vi "CRYTest Changing State.vi"(6 "Save?":bool, 8 "Origine Calibration":T1 {"Calibration 2D"."Sens Curve"."Z data" items=["dB", "Lin"]; "Calibration 2D"."Sens Curve"."X data" items=["dB", "Lin"]; "Calibration 2D"."Sens Curve"."Y data" items=["dB", "Lin"]; "Calibration 2D"."Sens Curve"."Z dB ref" format="%.1f"; "Calibration 2D"."Sens Curve"."Z axis" items=["Log", "Lin"]; "Calibration 2D"."Sens Curve"."X dB ref" format="%.1f"; "Calibration 2D"."Sens Curve"."X axis" items=["Log", "Lin"]; "Calibration 2D"."Sens Curve"."Y axis" items=["Log", "Lin"]; "Calibration 2D"."Sens Curve"."Y dB ref" format="%.1f"; "Calibration 2D"."Sens Curve"."Curve"."z" format="%.2f"; "Calibration 2D"."Sens Curve"."Curve"."y" format="%.2p"; "Calibration 2D"."Sens Curve"."Curve"."x" format="%.2f"; "Calibration 2D"."EQ Curve"."Z data" items=["dB", "Lin"]; "Calibration 2D"."EQ Curve"."X data" items=["dB", "Lin"]; "Calibration 2D"."EQ Curve"."Y data" items=["dB", "Lin"]; "Calibration 2D"."EQ Curve"."Z dB ref" format="%.1f"; "Calibration 2D"."EQ Curve"."Z axis" items=["Log", "Lin"]; "Calibration 2D"."EQ Curve"."X dB ref" format="%.1f"; "Calibration 2D"."EQ Curve"."X axis" items=["Log", "Lin"]; "Calibration 2D"."EQ Curve"."Y axis" items=["Log", "Lin"]; "Calibration 2D"."EQ Curve"."Y dB ref" format="%.1f"; "Calibration 2D"."EQ Curve"."Curve"."z" format="%.2f"; "Calibration 2D"."EQ Curve"."Curve"."y" format="%.2f"; "Calibration 2D"."EQ Curve"."Curve"."x" format="%.2f"; "Calibration 2D"."Corr Curve"."Z data" items=["dB", "Lin"]; "Calibration 2D"."Corr Curve"."X data" items=["dB", "Lin"]; "Calibration 2D"."Corr Curve"."Y data" items=["dB", "Lin"]; "Calibration 2D"."Corr Curve"."Z dB ref" format="%.1f"; "Calibration 2D"."Corr Curve"."Z axis" items=["Log", "Lin"]; "Calibration 2D"."Corr Curve"."X dB ref" format="%.1f"; "Calibration 2D"."Corr Curve"."X axis" items=["Log", "Lin"]; "Calibration 2D"."Corr Curve"."Y axis" items=["Log", "Lin"]; "Calibration 2D"."Corr Curve"."Y dB ref" format="%.1f"; "Calibration 2D"."Corr Curve"."Curve"."z" format="%.2f"; "Calibration 2D"."Corr Curve"."Curve"."y" format="%.2f"; "Calibration 2D"."Corr Curve"."Curve"."x" format="%.2f"; "Calibration 2D"."Calibration"."EQ Step size" items=["R10", "R20", "R40", "R80", "User"]; "Calibration 2D"."Calibration"."Corr Step size" items=["R10", "R20", "R40", "R80", "User"]}, 9 "New Calibration":T1 {"Calibration 2D"."Sens Curve"."Z data" items=["dB", "Lin"]; "Calibration 2D"."Sens Curve"."X data" items=["dB", "Lin"]; "Calibration 2D"."Sens Curve"."Y data" items=["dB", "Lin"]; "Calibration 2D"."Sens Curve"."Z dB ref" format="%.1f"; "Calibration 2D"."Sens Curve"."Z axis" items=["Log", "Lin"]; "Calibration 2D"."Sens Curve"."X dB ref" format="%.1f"; "Calibration 2D"."Sens Curve"."X axis" items=["Log", "Lin"]; "Calibration 2D"."Sens Curve"."Y axis" items=["Log", "Lin"]; "Calibration 2D"."Sens Curve"."Y dB ref" format="%.1f"; "Calibration 2D"."Sens Curve"."Curve"."z" format="%.2f"; "Calibration 2D"."Sens Curve"."Curve"."y" format="%.2p"; "Calibration 2D"."Sens Curve"."Curve"."x" format="%.2f"; "Calibration 2D"."EQ Curve"."Z data" items=["dB", "Lin"]; "Calibration 2D"."EQ Curve"."X data" items=["dB", "Lin"]; "Calibration 2D"."EQ Curve"."Y data" items=["dB", "Lin"]; "Calibration 2D"."EQ Curve"."Z dB ref" format="%.1f"; "Calibration 2D"."EQ Curve"."Z axis" items=["Log", "Lin"]; "Calibration 2D"."EQ Curve"."X dB ref" format="%.1f"; "Calibration 2D"."EQ Curve"."X axis" items=["Log", "Lin"]; "Calibration 2D"."EQ Curve"."Y axis" items=["Log", "Lin"]; "Calibration 2D"."EQ Curve"."Y dB ref" format="%.1f"; "Calibration 2D"."EQ Curve"."Curve"."z" format="%.2f"; "Calibration 2D"."EQ Curve"."Curve"."y" format="%.2f"; "Calibration 2D"."EQ Curve"."Curve"."x" format="%.2f"; "Calibration 2D"."Corr Curve"."Z data" items=["dB", "Lin"]; "Calibration 2D"."Corr Curve"."X data" items=["dB", "Lin"]; "Calibration 2D"."Corr Curve"."Y data" items=["dB", "Lin"]; "Calibration 2D"."Corr Curve"."Z dB ref" format="%.1f"; "Calibration 2D"."Corr Curve"."Z axis" items=["Log", "Lin"]; "Calibration 2D"."Corr Curve"."X dB ref" format="%.1f"; "Calibration 2D"."Corr Curve"."X axis" items=["Log", "Lin"]; "Calibration 2D"."Corr Curve"."Y axis" items=["Log", "Lin"]; "Calibration 2D"."Corr Curve"."Y dB ref" format="%.1f"; "Calibration 2D"."Corr Curve"."Curve"."z" format="%.2f"; "Calibration 2D"."Corr Curve"."Curve"."y" format="%.2f"; "Calibration 2D"."Corr Curve"."Curve"."x" format="%.2f"; "Calibration 2D"."Calibration"."EQ Step size" items=["R10", "R20", "R40", "R80", "User"]; "Calibration 2D"."Calibration"."Corr Step size" items=["R10", "R20", "R40", "R80", "User"]}, 10 "Signal Type":string, 11 "In/Out?":bool) -> (1 "Calibration 2D Cluster":T2={"Calibration"={"Calibration Step Name"="", "Device"="", "Correction Curve Name"="", "Equalization Curve Name"="", "Sensitivity Curve Name"="", "Corr Folder and File"="", "EQ Folder and File"="", "Sens Folder and File"="", "Corr Step size"=0, "EQ Step size"=0, "Input"=FALSE, "Last Cal Date (sec)"=timestamp(0 s since 1904-01-01), "Cha Name"="", "Corr Curve Found"=FALSE, "EQ Curve Found"=FALSE, "Sens Curve Found"=FALSE, "Signal Type"="", "Calibrated Device"="", "Hz"=0}, "Corr Curve"={"Name"="", "Curve"=[], "X data"=1, "Y data"=1, "Z data"=1, "X axis"=0, "Y axis"=1, "Z axis"=1, "X unit"="Hz", "Y unit"="", "Z unit"="deg.", "X dB ref"=1.0, "Y dB ref"=1.0, "Z dB ref"=1.0, "single val"=FALSE, "protected"=FALSE, "display X"=TRUE, "display Y"=TRUE, "display Z"=TRUE, "Test Info"="", "Step No."=0, "Plot Settings"={"Color"=0, "Interpolation"=0, "Point Style"=0, "Line Style"=0, "Point Color"=0, "Line Width"=0, "Bar Plot Style"=0, "Fill To"=0}, "AutoProtect"=FALSE}, "EQ Curve"={"Name"="", "Curve"=[], "X data"=1, "Y data"=1, "Z data"=1, "X axis"=0, "Y axis"=1, "Z axis"=1, "X unit"="Hz", "Y unit"="", "Z unit"="deg.", "X dB ref"=1.0, "Y dB ref"=1.0, "Z dB ref"=1.0, "single val"=FALSE, "protected"=FALSE, "display X"=TRUE, "display Y"=TRUE, "display Z"=TRUE, "Test Info"="", "Step No."=0, "Plot Settings"={"Color"=0, "Interpolation"=0, "Point Style"=0, "Line Style"=0, "Point Color"=0, "Line Width"=0, "Bar Plot Style"=0, "Fill To"=0}, "AutoProtect"=FALSE}, "Sens Curve"={"Name"="", "Curve"=[], "X data"=1, "Y data"=1, "Z data"=1, "X axis"=0, "Y axis"=1, "Z axis"=1, "X unit"="Hz", "Y unit"="", "Z unit"="deg.", "X dB ref"=1.0, "Y dB ref"=1.0, "Z dB ref"=1.0, "single val"=FALSE, "protected"=FALSE, "display X"=TRUE, "display Y"=TRUE, "display Z"=TRUE, "Test Info"="", "Step No."=0, "Plot Settings"={"Color"=0, "Interpolation"=0, "Point Style"=0, "Line Style"=0, "Point Color"=0, "Line Width"=0, "Bar Plot Style"=0, "Fill To"=0}, "AutoProtect"=FALSE}} {"Sens Curve"."Z data" items=["dB", "Lin"]; "Sens Curve"."X data" items=["dB", "Lin"]; "Sens Curve"."Y data" items=["dB", "Lin"]; "Sens Curve"."Z dB ref" format="%.1f"; "Sens Curve"."Z axis" items=["Log", "Lin"]; "Sens Curve"."X dB ref" format="%.1f"; "Sens Curve"."X axis" items=["Log", "Lin"]; "Sens Curve"."Y axis" items=["Log", "Lin"]; "Sens Curve"."Y dB ref" format="%.1f"; "Sens Curve"."Curve"."z" format="%.2f"; "Sens Curve"."Curve"."y" format="%.2f"; "Sens Curve"."Curve"."x" format="%.2f"; "EQ Curve"."Z data" items=["dB", "Lin"]; "EQ Curve"."X data" items=["dB", "Lin"]; "EQ Curve"."Y data" items=["dB", "Lin"]; "EQ Curve"."Z dB ref" format="%.1f"; "EQ Curve"."Z axis" items=["Log", "Lin"]; "EQ Curve"."X dB ref" format="%.1f"; "EQ Curve"."X axis" items=["Log", "Lin"]; "EQ Curve"."Y axis" items=["Log", "Lin"]; "EQ Curve"."Y dB ref" format="%.1f"; "EQ Curve"."Curve"."z" format="%.2f"; "EQ Curve"."Curve"."y" format="%.2f"; "EQ Curve"."Curve"."x" format="%.2f"; "Corr Curve"."Z data" items=["dB", "Lin"]; "Corr Curve"."X data" items=["dB", "Lin"]; "Corr Curve"."Y data" items=["dB", "Lin"]; "Corr Curve"."Z dB ref" format="%.1f"; "Corr Curve"."Z axis" items=["Log", "Lin"]; "Corr Curve"."X dB ref" format="%.1f"; "Corr Curve"."X axis" items=["Log", "Lin"]; "Corr Curve"."Y axis" items=["Log", "Lin"]; "Corr Curve"."Y dB ref" format="%.1f"; "Corr Curve"."Curve"."z" format="%.2f"; "Corr Curve"."Curve"."y" format="%.2f"; "Corr Curve"."Curve"."x" format="%.2f"; "Calibration"."EQ Step size" items=["R10", "R20", "R40", "R80", "User"]; "Calibration"."Corr Step size" items=["R10", "R20", "R40", "R80", "User"]}, 2 "Changed/Added":bool, 3 "Index":i32)   [LabVIEW 2013]
uses:
  Typedef Control/CRYCalibration All Cluster.ctl
  Typedef Control/CRYCalibration 2DCluster.ctl
  Typedef Control/CRYCalibration Cluster.ctl
  Typedef Control/CRYData Cluster.ctl
  CRYProject/CRYProject Editor Global.vi
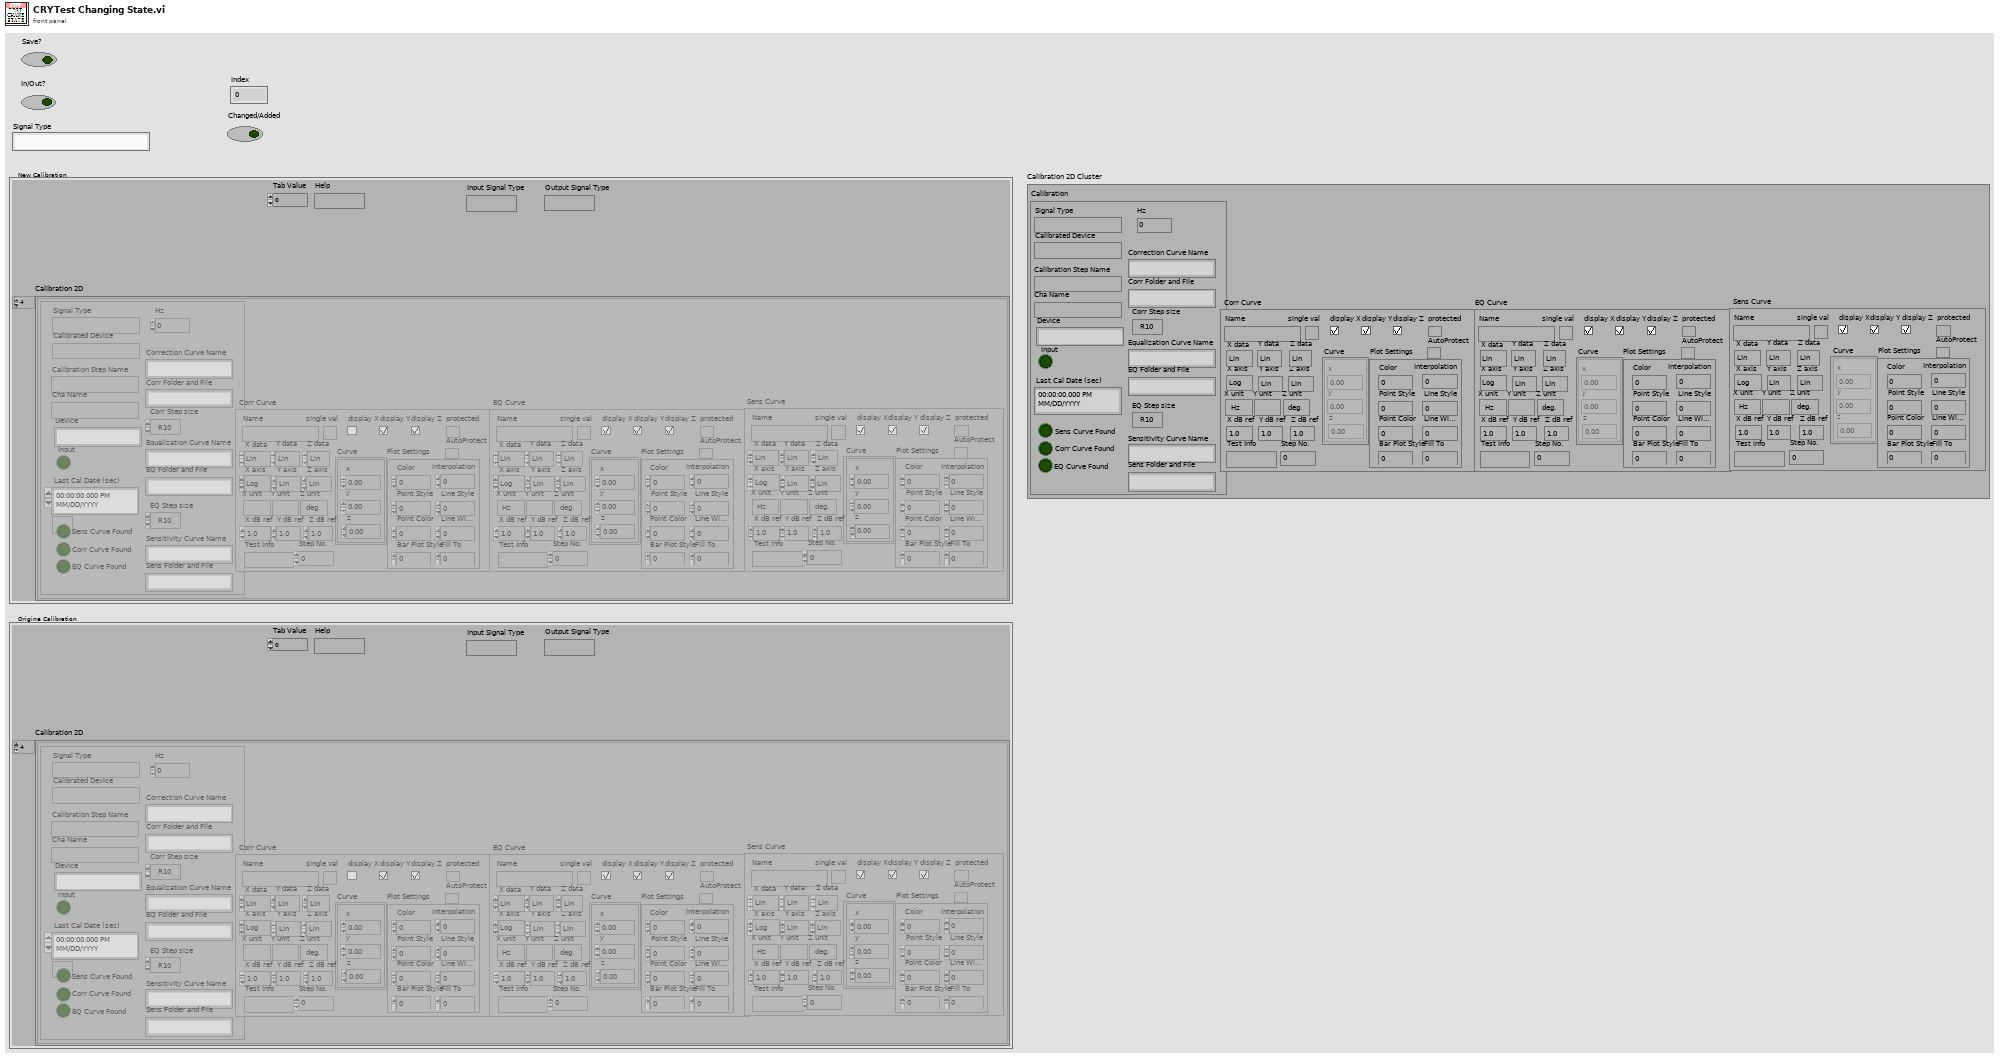
[diagram p1: front panel]
types:
  T1 = typedef "CRYCalibration All Cluster.ctl" = cluster{"Calibration 2D":T2[], "Help":string, "Tab Value":i32, "Input Signal Type":string, "Output Signal Type":string}
  T2 = typedef "CRYCalibration 2DCluster.ctl" = cluster{"Calibration":T3, "Corr Curve":T4, "EQ Curve":T4, "Sens Curve":T4}
  T3 = typedef "CRYCalibration Cluster.ctl" = cluster{"Calibration Step Name":string, "Device":string, "Correction Curve Name":string, "Equalization Curve Name":string, "Sensitivity Curve Name":string, "Corr Folder and File":string, "EQ Folder and File":string, "Sens Folder and File":string, "Corr Step size":u16, "EQ Step size":u16, "Input":bool, "Last Cal Date (sec)":timestamp, "Cha Name":string, "Corr Curve Found":bool, "EQ Curve Found":bool, "Sens Curve Found":bool, "Signal Type":string, "Calibrated Device":string, "Hz":u32}
  T4 = typedef "CRYData Cluster.ctl" = cluster{"Name":string, "Curve":cluster{"x":dbl, "y":dbl, "z":dbl}[], "X data":u16, "Y data":u16, "Z data":u16, "X axis":u16, "Y axis":u16, "Z axis":u16, "X unit":string, "Y unit":string, "Z unit":string, "X dB ref":dbl, "Y dB ref":dbl, "Z dB ref":dbl, "single val":bool, "protected":bool, "display X":bool, "display Y":bool, "display Z":bool, "Test Info":string, "Step No.":i32, "Plot Settings":cluster{"Color":u32, "Interpolation":u8, "Point Style":u8, "Line Style":u8, "Point Color":u32, "Line Width":u8, "Bar Plot Style":u8, "Fill To":i16}, "AutoProtect":bool}
  T5 = typedef "CRYStep.ctl" = cluster{"No.VI":i32, "Category":string, "StepName":string, "Seq setup flattened":string, "Comment":string, "Steps config.":bool[], "Jump config":i32[], "Start":dbl, "Increment":dbl, "Name":string, "Unit":string, "Y data":u16, "Y prefix":string, "Y dB ref":dbl, "Y unit":string, "Repeat State Array":cluster{"Start":dbl, "Increment":dbl, "Count":i32, "Num":i32}[]}
  T6 = cluster{"Calibration":cluster{"Calibration Step Name":bool, "Device":bool, "Correction Curve Name":bool, "Equalization Curve Name":bool, "Sensitivity Curve Name":bool, "Corr Folder and File":bool, "EQ Folder and File":bool, "Sens Folder and File":bool, "Corr Step size":bool, "EQ Step size":bool, "Input":bool, "Last Cal Date (sec)":bool, "Cha Name":bool, "Corr Curve Found":bool, "EQ Curve Found":bool, "Sens Curve Found":bool, "Signal Type":bool, "Calibrated Device":bool, "Hz":bool}, "Corr Curve":cluster{"Name":bool, "Curve":cluster{"x":bool, "y":bool, "z":bool}[], "X data":bool, "Y data":bool, "Z data":bool, "X axis":bool, "Y axis":bool, "Z axis":bool, "X unit":bool, "Y unit":bool, "Z unit":bool, "X dB ref":bool, "Y dB ref":bool, "Z dB ref":bool, "single val":bool, "protected":bool, "display X":bool, "display Y":bool, "display Z":bool, "Test Info":bool, "Step No.":bool, "Plot Settings":cluster{"Color":bool, "Interpolation":bool, "Point Style":bool, "Line Style":bool, "Point Color":bool, "Line Width":bool, "Bar Plot Style":bool, "Fill To":bool}, "AutoProtect":bool}, "EQ Curve":cluster{"Name":bool, "Curve":cluster{"x":bool, "y":bool, "z":bool}[], "X data":bool, "Y data":bool, "Z data":bool, "X axis":bool, "Y axis":bool, "Z axis":bool, "X unit":bool, "Y unit":bool, "Z unit":bool, "X dB ref":bool, "Y dB ref":bool, "Z dB ref":bool, "single val":bool, "protected":bool, "display X":bool, "display Y":bool, "display Z":bool, "Test Info":bool, "Step No.":bool, "Plot Settings":cluster{"Color":bool, "Interpolation":bool, "Point Style":bool, "Line Style":bool, "Point Color":bool, "Line Width":bool, "Bar Plot Style":bool, "Fill To":bool}, "AutoProtect":bool}, "Sens Curve":cluster{"Name":bool, "Curve":cluster{"x":bool, "y":bool, "z":bool}[], "X data":bool, "Y data":bool, "Z data":bool, "X axis":bool, "Y axis":bool, "Z axis":bool, "X unit":bool, "Y unit":bool, "Z unit":bool, "X dB ref":bool, "Y dB ref":bool, "Z dB ref":bool, "single val":bool, "protected":bool, "display X":bool, "display Y":bool, "display Z":bool, "Test Info":bool, "Step No.":bool, "Plot Settings":cluster{"Color":bool, "Interpolation":bool, "Point Style":bool, "Line Style":bool, "Point Color":bool, "Line Width":bool, "Bar Plot Style":bool, "Fill To":bool}, "AutoProtect":bool}}
  T7 = cluster{"Calibration Step Name":bool, "Device":bool, "Correction Curve Name":bool, "Equalization Curve Name":bool, "Sensitivity Curve Name":bool, "Corr Folder and File":bool, "EQ Folder and File":bool, "Sens Folder and File":bool, "Corr Step size":bool, "EQ Step size":bool, "Input":bool, "Last Cal Date (sec)":bool, "Cha Name":bool, "Corr Curve Found":bool, "EQ Curve Found":bool, "Sens Curve Found":bool, "Signal Type":bool, "Calibrated Device":bool, "Hz":bool}
  T8 = cluster{"Name":bool, "Curve":cluster{"x":bool, "y":bool, "z":bool}[], "X data":bool, "Y data":bool, "Z data":bool, "X axis":bool, "Y axis":bool, "Z axis":bool, "X unit":bool, "Y unit":bool, "Z unit":bool, "X dB ref":bool, "Y dB ref":bool, "Z dB ref":bool, "single val":bool, "protected":bool, "display X":bool, "display Y":bool, "display Z":bool, "Test Info":bool, "Step No.":bool, "Plot Settings":cluster{"Color":bool, "Interpolation":bool, "Point Style":bool, "Line Style":bool, "Point Color":bool, "Line Width":bool, "Bar Plot Style":bool, "Fill To":bool}, "AutoProtect":bool}
  T9 = cluster{"Name":bool, "Curve":cluster{"x":bool, "y":bool, "z":bool}[], "X data":bool, "Y data":bool, "Z data":bool, "X axis":bool, "Y axis":bool, "Z axis":bool, "X unit":bool, "Y unit":bool, "Z unit":bool, "X dB ref":bool, "Y dB ref":bool, "Z dB ref":bool, "single val":bool, "protected":bool, "display X":bool, "display Y":bool, "display Z":bool, "Test Info":bool, "Step No.":bool, "Plot Settings":cluster{"Color":bool, "Interpolation":bool, "Point Style":bool, "Line Style":bool, "Point Color":bool, "Line Width":bool, "Bar Plot Style":bool, "Fill To":bool}, "AutoProtect":bool}[]
  T10 = cluster{"Color":bool, "Interpolation":bool, "Point Style":bool, "Line Style":bool, "Point Color":bool, "Line Width":bool, "Bar Plot Style":bool, "Fill To":bool}
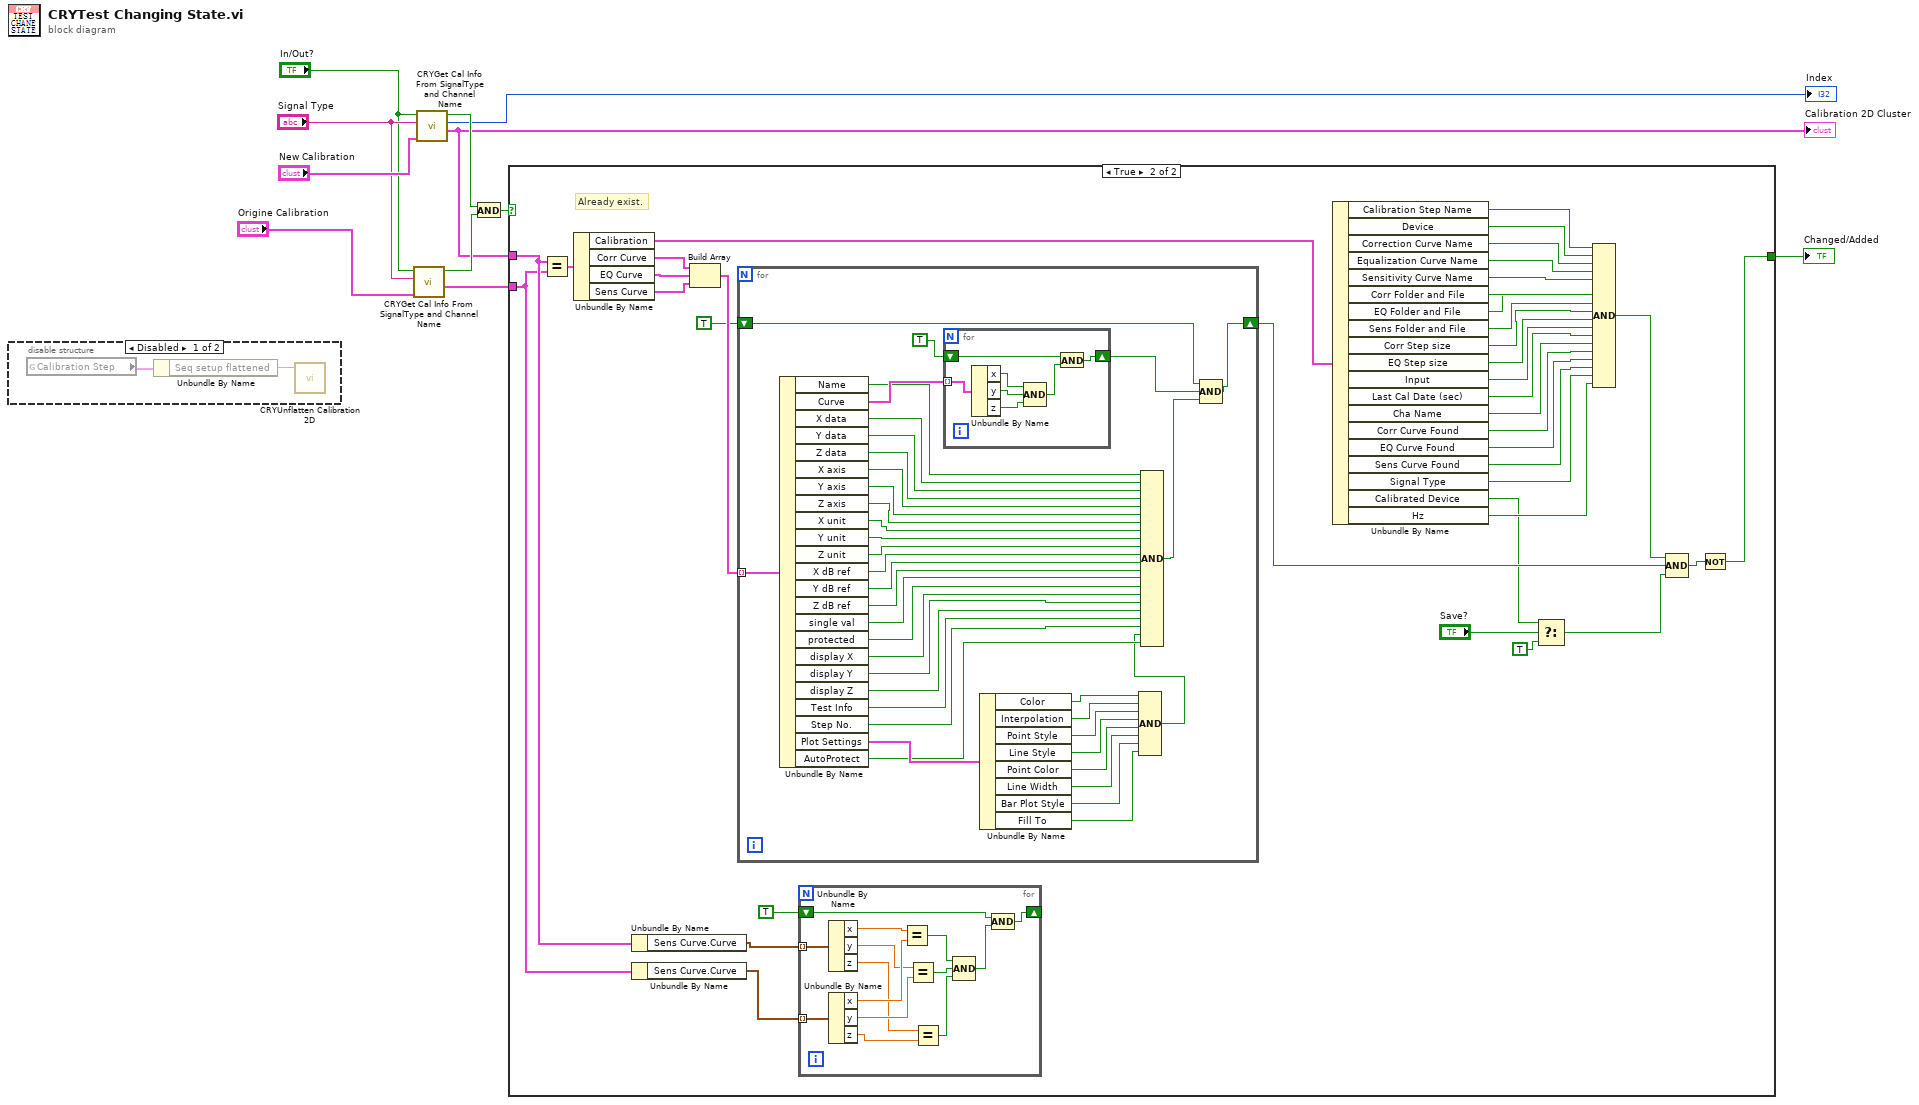
[diagram p0: block diagram]
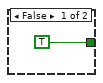
[diagram p3: hidden frame]
diagram:
  n1 = disable-structure shown="Disabled" {
    frame Disabled {
      n2 = global read "CRYProject Editor Global.vi" "Calibration Step"() -> (w13:T5)
      n3 = Unbundle By Name(w13) -> ("Seq setup flattened"=w12:string)
      n4 = call "CRYUnflatten Calibration 2D.vi"("Flattened Calibration"=w12) -> ()  [unwired: 8 in, 3 out]
    }
    frame Enabled {
    }
  }
  n5 = call "CRYGet Cal Info From SignalType and Channel Name.vi"("Calibration"="Origine Calibration", "Signal Type"="Signal Type", "In/Out?"="In/Out?") -> ("Calibration 2D Cluster"=w3:T2, "Exist"=w7:bool)  [unwired: 6 in, 1 out]
  n6 = call "CRYGet Cal Info From SignalType and Channel Name.vi"("Calibration"="New Calibration", "Signal Type"="Signal Type", "In/Out?"="In/Out?") -> ("Calibration 2D Cluster"=w2:T2, "Index"=→"Index":i32, "Exist"=w8:bool)  [unwired: 6 in]
  "Calibration 2D Cluster" <- w2
  n7 = And(x=w8, y=w7) -> (x .and. y?=w6:bool)
  n8 = case shown="True" w6 {
    tunnel: [TRUE ("Changed") w25] -> w5
    tunnel: w3 -> [_ w22]
    tunnel: w2 -> [_ w23]
    frame False {
    }
    frame True {
      # "Already exist."
      n9 = Equal?(x=w23, y=w22) -> (x = y?=w52:T6)
      n10 = Unbundle By Name(w52) -> ("Calibration"=w51:T7, "Corr Curve"=w50:T8, "EQ Curve"=w49:T8, "Sens Curve"=w24:T8)
      n11 = Unbundle By Name(w23) -> ("Sens Curve.Curve"=w21:cluster{"x":dbl, "y":dbl, "z":dbl}[])
      n12 = Unbundle By Name(w22) -> ("Sens Curve.Curve"=w20:cluster{"x":dbl, "y":dbl, "z":dbl}[])
      n13 = Build Array(w50, w49, w24) -> (w48:T9)
      n14 = for {
        tunnel: w48 -> [w104] mode=indexing
        shift-right: [w68] -> w27
        shift-left: TRUE ("Name") -> [w71]
        n15 = Unbundle By Name(w104) -> ("Name"=w100:bool, "Curve"=w103:cluster{"x":bool, "y":bool, "z":bool}[], "X data"=w99:bool, "Y data"=w98:bool, "Z data"=w97:bool, "X axis"=w96:bool, "Y axis"=w95:bool, "Z axis"=w94:bool, "X unit"=w93:bool, "Y unit"=w92:bool, "Z unit"=w91:bool, "X dB ref"=w90:bool, "Y dB ref"=w89:bool, "Z dB ref"=w88:bool, "single val"=w87:bool, "protected"=w86:bool, "display X"=w85:bool, "display Y"=w84:bool, "display Z"=w83:bool, "Test Info"=w82:bool, "Step No."=w81:bool, "Plot Settings"=w101:T10, "AutoProtect"=w80:bool)
        n16 = for {
          tunnel: w103 -> [w111] mode=indexing
          shift-right: [w105] -> w70
          shift-left: TRUE ("Name") -> [w107]
          n17 = Unbundle By Name(w111) -> ("x"=w110:bool, "y"=w109:bool, "z"=w108:bool)
          n18 = Compound Arithmetic op=AND(w110, w109, w108) -> (w106:bool)
          n19 = And(x=w107, y=w106) -> (x .and. y?=w105:bool)
        }
        n20 = Unbundle By Name(w101) -> ("Color"=w79:bool, "Interpolation"=w78:bool, "Point Style"=w77:bool, "Line Style"=w76:bool, "Point Color"=w75:bool, "Line Width"=w74:bool, "Bar Plot Style"=w73:bool, "Fill To"=w72:bool)
        n21 = Compound Arithmetic op=AND(w79, w78, w77, w76, w75, w74, w73, w72) -> (w67:bool)
        n22 = Compound Arithmetic op=AND(w100, w99, w98, w97, w96, w95, w94, w93, w92, w91, w90, w89, w88, w87, w86, w85, w84, w83, w82, w81, w67, w80) -> (w69:bool)
        n23 = Compound Arithmetic op=AND(w71, w70, w69) -> (w68:bool)
      }
      n24 = for {
        tunnel: w21 -> [w66] mode=indexing
        tunnel: w20 -> [w65] mode=indexing
        shift-right: [w53] -> _
        shift-left: TRUE ("Name") -> [w54]
        n25 = Unbundle By Name(w66) -> ("x"=w64:dbl, "y"=w62:dbl, "z"=w59:dbl)
        n26 = Unbundle By Name(w65) -> ("x"=w63:dbl, "y"=w61:dbl, "z"=w60:dbl)
        n27 = Equal?(x=w64, y=w63) -> (x = y?=w58:bool)
        n28 = Equal?(x=w62, y=w61) -> (x = y?=w57:bool)
        n29 = Equal?(x=w59, y=w60) -> (x = y?=w56:bool)
        n30 = Compound Arithmetic op=AND(w58, w57, w56) -> (w55:bool)
        n31 = Compound Arithmetic op=AND(w54, w55) -> (w53:bool)
      }
      n32 = Unbundle By Name(w51) -> ("Calibration Step Name"=w46:bool, "Device"=w45:bool, "Correction Curve Name"=w44:bool, "Equalization Curve Name"=w43:bool, "Sensitivity Curve Name"=w42:bool, "Corr Folder and File"=w41:bool, "EQ Folder and File"=w40:bool, "Sens Folder and File"=w39:bool, "Corr Step size"=w38:bool, "EQ Step size"=w37:bool, "Input"=w36:bool, "Last Cal Date (sec)"=w35:bool, "Cha Name"=w34:bool, "Corr Curve Found"=w33:bool, "EQ Curve Found"=w32:bool, "Sens Curve Found"=w31:bool, "Signal Type"=w30:bool, "Calibrated Device"=w17:bool, "Hz"=w29:bool)
      n33 = Select(t=w17, s="Save?", f=TRUE) -> (s? t:f=w16:bool)
      n34 = Compound Arithmetic op=AND(w46, w45, w44, w43, w42, w41, w40, w39, w38, w37, w36, w35, w34, w33, w32, w31, w30, w29) -> (w28:bool)
      n35 = Compound Arithmetic op=AND(w28, w27, w16) -> (w26:bool)
      n36 = Not(x=w26) -> (.not. x?=w25:bool)
    }
  }
  "Changed/Added" <- w5
